vi "Set Termination.vi"(0 "Tosca in":refnum<class "Parameters.lvclass">, 5 "Termination":refnum<class "Termination.lvclass"> caption="Timeout", 7 "stateIndex":i32, 9 "termIndex":i32, 11 "error in (no error)":errorcluster) -> (4 "Tosca out":refnum<class "Parameters.lvclass">, 8 "change action state":i32, 10 "TTL-only":bool, 15 "error out":errorcluster)   [LabVIEW 2015, in "Parameters.lvclass"]
uses:
  Parameters.lvclass
  Termination/Termination.lvclass
  Parameters.lvclass/Parameters.ctl
  Termination/Termination.lvclass/Termination.ctl
  State/State.lvclass/State.ctl
  Termination/Read Link to.vi
  Termination/Read Action.vi
  State/Read TTL-only.vi
  State/State.lvclass
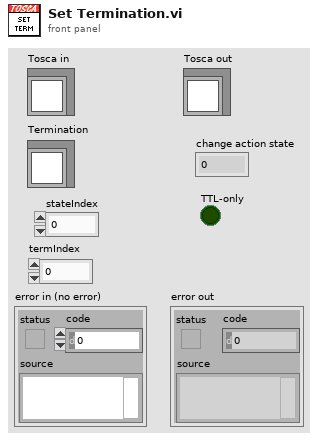
[diagram p1: front panel]
types:
  T1 = typedef "Tosca-Termination Condition Action.ctl" = enum16{"End state", "Complete state", "TTL only"}
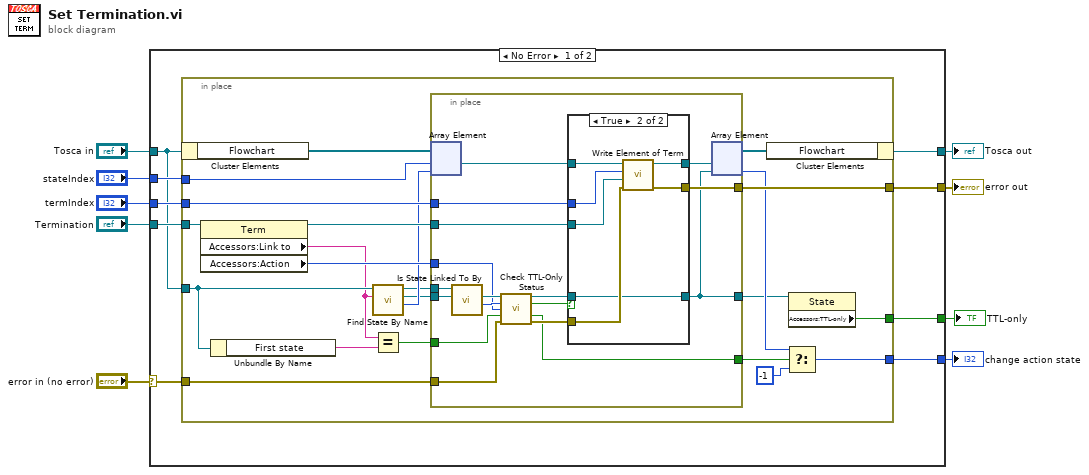
[diagram p0: block diagram]
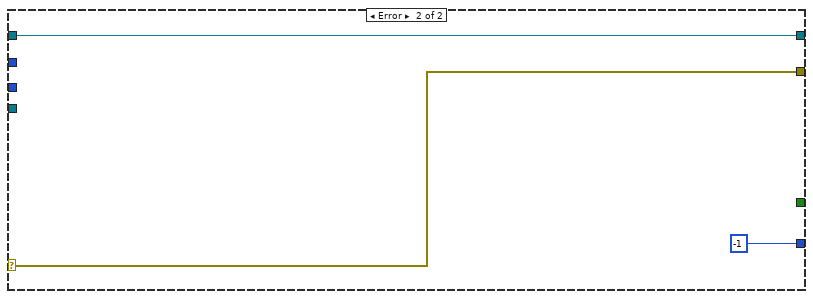
[diagram p3: hidden frame]
diagram:
  n1 = case shown="No Error" "error in (no error)" {
    selector: "error in (no error)" -> [w14 w70]
    tunnel: [w13 w70] -> w8
    tunnel: [w18 w69] -> w6
    tunnel: "Tosca in" -> [w11 w69]
    tunnel: "stateIndex" -> [w17 _]
    tunnel: "termIndex" -> [w16 _]
    tunnel: "Termination" -> [w15 _]
    tunnel: [w12 -1] -> w2
    tunnel: [w10 _] -> w1
    frame No Error {
      n2 = in-place {
        in-place-border: w17 -> [w40]
        in-place-border: w15 -> [w35]
        in-place-border: w16 -> [w38]
        in-place-border: w14 -> [w37]
        in-place-border: [w36] -> w13
        in-place-border: [w25] -> w12
        in-place-border: w11 -> [w22]
        in-place-border: [w23] -> w10
        n3 = in-place-cluster #1(w11) -> ("Flowchart"=w32:refnum<class "State.lvclass">[])
        n4 = property class="Term"(reference=w35) -> (reference out=w34:refnum<class "Termination.lvclass">, "Accessors:Link to"=w21:string, "Accessors:Action"=w33:T1)  [unwired: 1 in, 1 out]
        n5 = Unbundle By Name(w22) -> ("First state"=w20:string)
        n6 = call "Find State By Name.vi"("Name"=w21, "Tosca in"=w22) -> ("Index"=w31:i32, "State"=w29:refnum<class "State.lvclass">, "Tosca out"=w30:refnum<class "Parameters.lvclass">)  [unwired: 6 in, 1 out]
        n7 = Equal?(x=w21, y=w20) -> (x = y?=w19:bool)
        n8 = in-place {
          in-place-border: w34 -> [w57]
          in-place-border: w38 -> [w55]
          in-place-border: w37 -> [w53]
          in-place-border: [w54] -> w36
          in-place-border: [w48] -> w28
          in-place-border: w33 -> [w47]
          in-place-border: w30 -> [w46]
          in-place-border: w29 -> [w45]
          in-place-border: [w42] -> w24
          in-place-border: w19 -> [w41]
          n9 = in-place-array #2(w32, w40, w31) -> (w44:refnum<class "State.lvclass">)  [unwired: 1 out]
          n10 = call "Is State Linked To By.vi"("State in"=w45, "Tosca in"=w46) -> ("number"=w51:i16, "State thru"=w52:refnum<class "State.lvclass">)  [unwired: 5 in, 3 out]
          n11 = call "Check TTL-Only Status.vi"("State in"=w52, "Num linking to this state"=w51, "Action"=w47, "Start state"=w41, "error in (no error)"=w53) -> ("State out"=w43:refnum<class "State.lvclass">, "accepted"=w49:bool, "TTL-only changed"=w48:bool, "error out"=w50:errorcluster)  [unwired: 7 in]
          n12 = case shown="True" w49 {
            tunnel: w57 -> [_ w67]
            tunnel: [w60 w66] -> w56
            tunnel: w55 -> [_ w65]
            tunnel: [w59 w64] -> w54
            tunnel: w44 -> [w60 w63]
            tunnel: w50 -> [w59 w62]
            tunnel: w43 -> [w58 w61]
            tunnel: [w58 w61] -> w42
            frame False {
            }
            frame True {
              n13 = call "Write Element of Term.vi"("error in (no error)"=w62, "Termination"=w67, "index"=w65, "State in"=w63) -> ("error out"=w64:errorcluster, "State out"=w66:refnum<class "State.lvclass">)  [unwired: 6 in]
            }
          }
          n14 = in-place-array #2(w56, w42) -> (w39:refnum<class "State.lvclass">[], w27:i32)  [unwired: 1 out]
        }
        n15 = in-place-cluster #1("Flowchart"=w39) -> (w18:refnum<class "Parameters.lvclass">)
        n16 = Select(t=w27, s=w28, f=-1) -> (s? t:f=w25:i32)
        n17 = property class="State"(reference=w24) -> ("Accessors:TTL-only"=w23:bool)  [unwired: 1 in, 2 out]
      }
    }
    frame Error {
    }
  }
  "error out" <- w8
  "Tosca out" <- w6
  "change action state" <- w2
  "TTL-only" <- w1
